vi "mfd_main.vi"   [LabVIEW 2023]
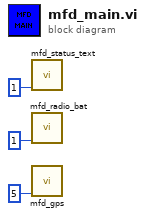
[diagram p0: block diagram]
diagram:
  n1 = call "mfd_status_text.vi"("Refresh Rate (Hz)"=u32 1) -> ()  [unwired: 11 in]
  n2 = call "mfd_radio_bat.vi"("Refresh Rate (Hz)"=u32 1) -> ()  [unwired: 11 in]
  n3 = call "mfd_gps.vi"("Refresh Rate (Hz)"=u32 5) -> ()  [unwired: 11 in]
